vi "Get_users_email_addresses.vi"(1 "OK":bool) -> ()   [LabVIEW 2017]
uses:
  File/Setup_Filetype.ctl
  Globals/Meas_global.vi
  Globals/Preference_global.vi
panel:
  out "Times Mon - Fri":string[](array[string])=["Midnight to 1am", "1am to 2am", "2am to 3am", "3am to 4am", "4am to 5am", "5am to 6am", "6am to 7am", "7am to 8am", "8am to 9am", "9am to 10am", "10am to 11am", "11am to Midday", "Midday to 1pm", "1pm to 2pm", "2pm to 3pm", "3pm to 4pm", "4pm to 5pm", "5pm to 6pm", "6pm to 7pm", "7pm to 8pm", "8pm to 9pm", "9pm to 10pm", "10pm to 11pm", "11pm to Midnight"]
  in  "SMS Action":bool[](array[boolean])=[TRUE, FALSE, TRUE]
  out "Message":string
  in  "Email addresses":string[](array[string])
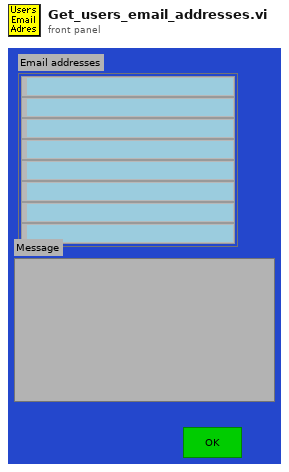
[diagram p1: front panel]
types:
  T1 = typedef "Setup_Filetype.ctl" = enum16{"Measurement Setups", "Calibration Setups", "General", "Results File Plotter Setups", "Speed Calib Tweaks"}
  T2 = enum16{"Highest", "High", "Normal", "Low", "Lowest"}
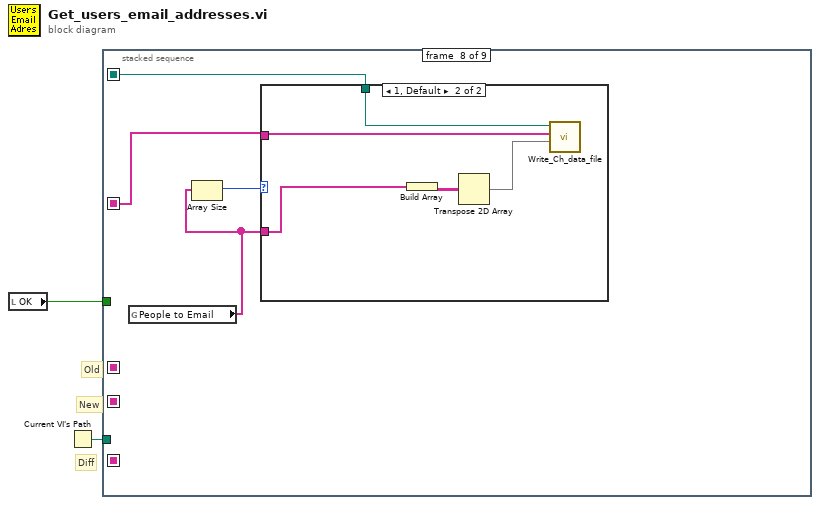
[diagram p0: block diagram]
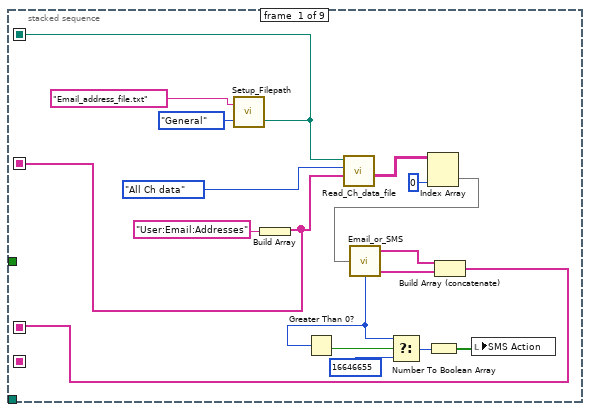
[diagram p2: hidden frame]
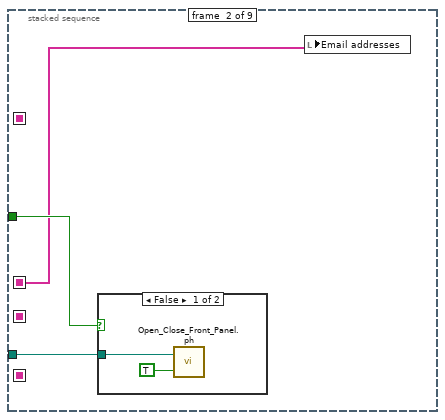
[diagram p3: hidden frame]
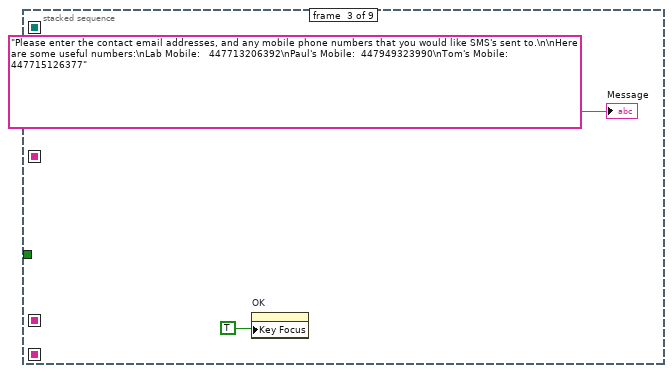
[diagram p5: hidden frame]
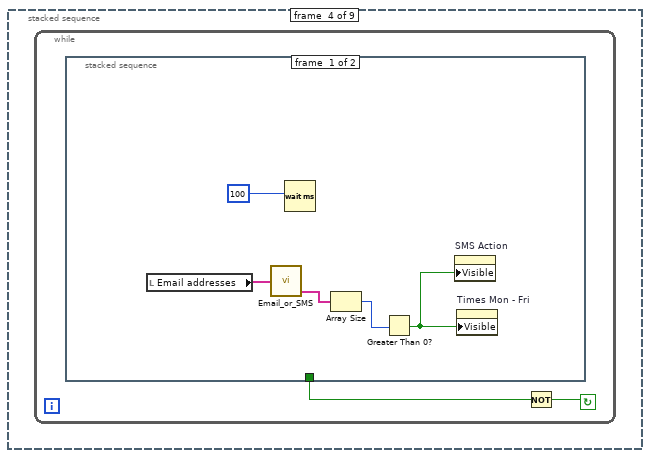
[diagram p6: hidden frame]
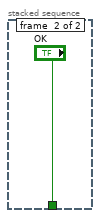
[diagram p7: hidden frame]
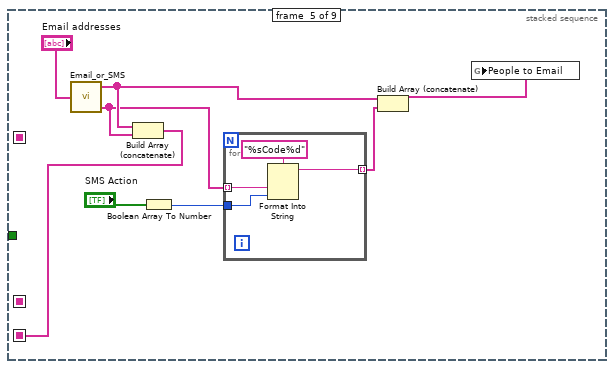
[diagram p8: hidden frame]
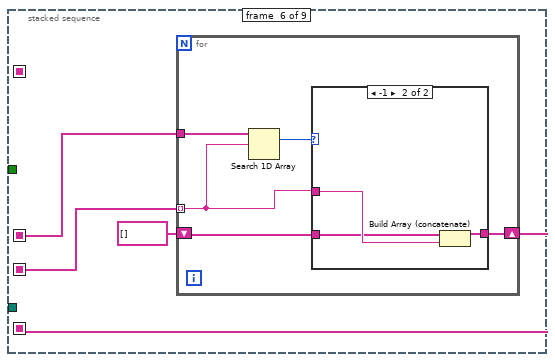
[diagram p9: hidden frame]
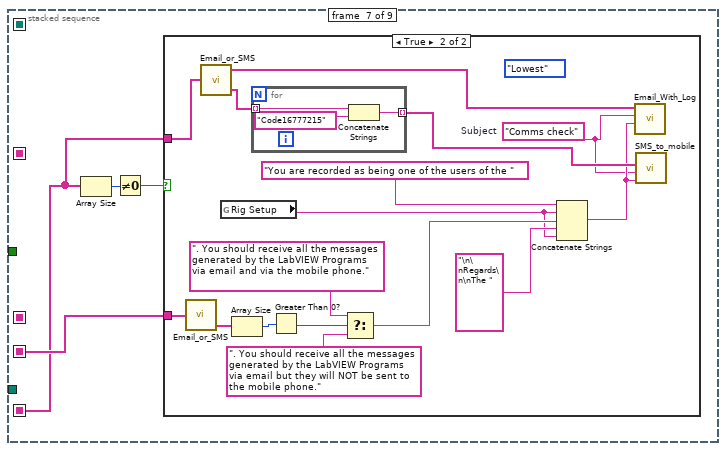
[diagram p11: hidden frame]
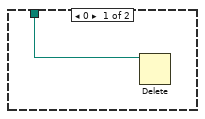
[diagram p13: hidden frame]
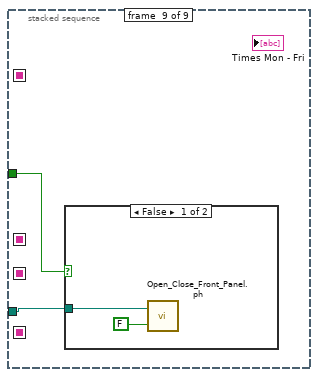
[diagram p14: hidden frame]
diagram:
  # "Diff"
  # "Old"
  # "New"
  n1 = local read "OK"() -> (w1:bool)
  n2 = Current VI's Path() -> (path=w2:path)
  n3 = stacked-sequence {
    seq-local: [_ _ _ _ w36 _ _ _ _] -> [_ _ _ _ _ w47 w62 _ _]
    seq-local: [w3 _ _ _ _ _ _ _ _] -> [_ _ _ _ _ _ _ w86 _]
    seq-local: [w16 _ _ _ _ _ _ _ _] -> [_ _ _ _ _ _ _ w85 _]
    seq-local: [w11 _ _ _ _ _ _ _ _] -> [_ w20 _ _ _ w50 _ _ _]
    seq-local: [_ _ _ _ _ w48 _ _ _] -> [_ _ _ _ _ _ w61 _ _]
    tunnel: w2 -> [_ w22 _ _ _ _ _ _ w94]
    tunnel: w1 -> [_ w21 _ _ _ _ _ _ w93]
    frame #0 {
      n4 = call "Setup_Filepath.vi"("Setup File Type"=Setup_Filetype."General", "Filename in"="Email_address_file.txt" ("Substring")) -> ("Filename Out"=w3:path)  [unwired: 1 out]
      n5 = Build Array("User:Email:Addresses") -> (w16:string[])
      n6 = call "Read_Ch_data_file.vi"("Present Channels"=w16, "Output"=enum16{"All Ch data", "The last few rows"}."All Ch data", "Filename"=w3) -> ("Channel Values"=w15:string[][])  [unwired: 2 in, 4 out]
      n7 = Index Array(array=w15, index (col)=0 ("Index")) -> (element=w14:string[])  [unwired: 1 in]
      n8 = call "Email_or_SMS.vi"("Email address"=w14) -> ("Send Code"=w9:u32, "Email"=w13:string[], "All Mobile Numbers"=w12:string[])  [unwired: 1 out]
      n9 = Greater Than 0?(x=w9) -> (x > 0?=w8:bool)
      n10 = Select(t=w9, s=w8, f=u32 16646655 ("number")) -> (s? t:f=w6:u32)
      n11 = Number To Boolean Array(number=w6) -> (Boolean array=w10:bool[])
      n12 = Build Array (concatenate)(w13, w12) -> (w11:string[])
      n13 = local write "SMS Action"(w10) -> ()
    }
    frame #1 {
      n14 = case shown="False" w21 {
        tunnel: w22 -> [w24 _]
        frame False {
          n15 = call "Open_Close_Front_Panel.ph.vi"("Front Panel Window:Open"=TRUE, "VI path"=w24) -> ()  [unwired: 2 out]
        }
        frame True {
        }
      }
      n16 = local write "Email addresses"(w20) -> ()
    }
    frame #2 {
      n17 = property on="OK" class="Bool (strict)"("Key Focus"=TRUE ("Write Attribute")) -> ()  [unwired: 2 in, 2 out]
      "Message" <- "Please enter the contact email addresses, and any mobile phone numbers that you would like SMS's sent to.\n\nHere are some useful numbers:\nLab Mobile:   447713206392\nPaul's Mobile:  447949323990\nTom's Mobile:  447715126377" ("Message")
    }
    frame #3 {
      n18 = while {
        stop <- w28 continue-if-true
        n19 = stacked-sequence {
          tunnel: [_ "OK"] -> w27
          frame #0 {
            n20 = local read "Email addresses"() -> (w32:string[])
            n21 = call "Email_or_SMS.vi"("Email address"=w32) -> ("All Mobile Numbers"=w31:string[])  [unwired: 3 out]
            n22 = Wait (ms)(milliseconds to wait=u32 100 ("milliseconds to Wait")) -> ()  [unwired: 1 out]
            n23 = Array Size(array=w31) -> (size(s)=w30:i32)
            n24 = Greater Than 0?(x=w30) -> (x > 0?=w29:bool)
            n25 = property on="SMS Action" class="Arr (strict)"("Visible"=w29) -> ()  [unwired: 2 in, 2 out]
            n26 = property on="Times Mon - Fri" class="Arr (strict)"("Visible"=w29) -> ()  [unwired: 2 in, 2 out]
          }
          frame #1 {
          }
        }
        n27 = Not(x=w27) -> (.not. x?=w28:bool)
      }
    }
    frame #4 {
      n28 = call "Email_or_SMS.vi"("Email address"="Email addresses") -> ("Email"=w38:string[], "All Mobile Numbers"=w37:string[])  [unwired: 2 out]
      n29 = Build Array (concatenate)(w38, w37) -> (w36:string[])
      n30 = Boolean Array To Number(Boolean array="SMS Action") -> (number=w40:u32)
      n31 = for {
        tunnel: w40 -> [w46]
        tunnel: w37 -> [w45] mode=indexing
        tunnel: [w43] -> w39 mode=indexing
        n32 = Format Into String(format string="%sCode%d" ("Format String"), w45, w46) -> (resulting string=w43:string)  [unwired: 2 in, 1 out]
      }
      n33 = Build Array (concatenate)(w38, w39) -> (w35:string[])
      n34 = global write "Meas_global.vi" "People to Email"(w35) -> ()
    }
    frame #5 {
      n35 = for {
        tunnel: w50 -> [w55]
        shift-right: [w52] -> w48
        shift-left: string[] [] -> [w53]
        tunnel: w47 -> [w51] mode=indexing
        n36 = Search 1D Array(1D array=w55, element=w51) -> (index of element=w54:i32)  [unwired: 1 out]
        n37 = case shown="-1" w54 {
          tunnel: w51 -> [_ w59]
          tunnel: w53 -> [w56 w58]
          tunnel: [w56 w57] -> w52
          frame 0, Default {
          }
          frame -1 {
            n38 = Build Array (concatenate)(w58, w59) -> (w57:string[])
          }
        }
      }
    }
    frame #6 {
      n39 = Array Size(array=w61) -> (size(s)=w63:i32)
      n40 = Not Equal To 0?(x=w63) -> (x != 0?=w60:bool)
      n41 = case shown="True" w60 {
        tunnel: w61 -> [_ w70]
        tunnel: w62 -> [_ w74]
        frame False {
        }
        frame True {
          (unwired) T2."Lowest" ("Priorities")
          w64 = "Comms check"  # Subject
          n42 = call "Email_or_SMS.vi"("Email address"=w74) -> ("All Mobile Numbers"=w73:string[])  [unwired: 3 out]
          n43 = call "Email_or_SMS.vi"("Email address"=w70) -> ("Email"=w69:string[], "All Mobile Numbers"=w68:string[])  [unwired: 2 out]
          n44 = global read "Preference_global.vi" "Rig Setup"() -> (w66:string)
          n45 = Array Size(array=w73) -> (size(s)=w72:i32)
          n46 = for {
            tunnel: w68 -> [w81] mode=indexing
            tunnel: [w80] -> w67 mode=indexing
            n47 = Concatenate Strings(w81, "Code16777215" ("Substring")) -> (w80:string)
          }
          n48 = Greater Than 0?(x=w72) -> (x > 0?=w71:bool)
          n49 = Select(t=". You should receive all the messages generated by the LabVIEW Programs via email and via the mobile phone." ("Message"), s=w71, f=". You should receive all the messages generated by the LabVIEW Programs via email but they will NOT be sent to the mobile phone." ("Message")) -> (s? t:f=w78:string)
          n50 = Concatenate Strings("You are recorded as being one of the users of the " ("Message"), w66, w78, "\n\nRegards\n\nThe " ("Message"), w66) -> (w65:string)
          n51 = call "Email_With_Log.vi"("recipients"=w69, "subject ([No Subject])"=w64, "message"=w65) -> ()  [unwired: 1 in, 3 out]
          n52 = call "SMS_to_mobile.vi"("SMS address"=w67, "Subject"=w64, "Message"=w65) -> ()  [unwired: 3 out]
        }
      }
    }
    frame #7 {
      n53 = global read "Meas_global.vi" "People to Email"() -> (w83:string[])
      n54 = Array Size(array=w83) -> (size(s)=w84:i32)
      n55 = case shown="1, Default" w84 {
        tunnel: w86 -> [w87 w92]
        tunnel: w85 -> [_ w91]
        tunnel: w83 -> [_ w88]
        frame 0 {
          n56 = Delete(path (use dialog)=w87) -> ()  [unwired: 1 in, 6 out]
        }
        frame 1, Default {
          n57 = Build Array(w88) -> (w90:string[][])
          n58 = Transpose 2D Array(2D array=w90) -> (transposed array=w89:string[][])
          n59 = call "Write_Ch_data_file.vi"("Channel Values"=w89, "Channel names"=w91, "Filename"=w92) -> ()  [unwired: 5 in, 4 out]
        }
      }
    }
    frame #8 {
      n60 = case shown="False" w93 {
        tunnel: w94 -> [w95 _]
        frame False {
          n61 = call "Open_Close_Front_Panel.ph.vi"("Front Panel Window:Open"=FALSE, "VI path"=w95) -> ()  [unwired: 2 out]
        }
        frame True {
        }
      }
    }
  }
